vi "User_Get_Auth_Code.vi"(8 "error in (no error)":errorcluster, 11 "URL In":string) -> (0 "error out":errorcluster, 3 "Auth Code":string)   [LabVIEW 2016]
uses:
  <vilib>/Platform/browser.llb/Open URL in Default Browser (string).vi
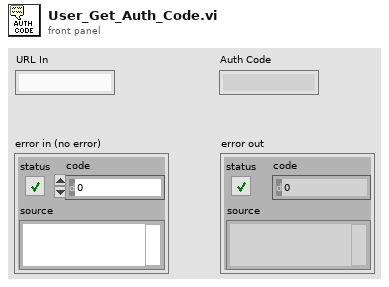
[diagram p1: front panel]
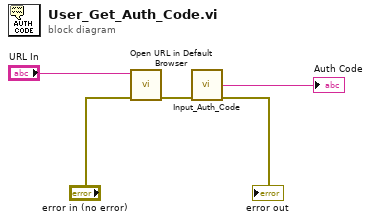
[diagram p0: block diagram]
diagram:
  n1 = call-poly <vilib>:"Open URL in Default Browser.vi"("error in (no error)"="error in (no error)", "URL"="URL In") -> ("error out"=→"error out":errorcluster)  [unwired: 4 in, 1 out]
  n2 = call "Input_Auth_Code.vi"() -> ("Code Out"=→"Auth Code":string)  [unwired: 1 in]
